vi "GetWinScale.vi"(8 "Error In":errorcluster, 11 "Window Name":string) -> (0 "Error Out":errorcluster, 3 "Scale":dbl)   [LabVIEW 2025]
uses:
  user32.dll
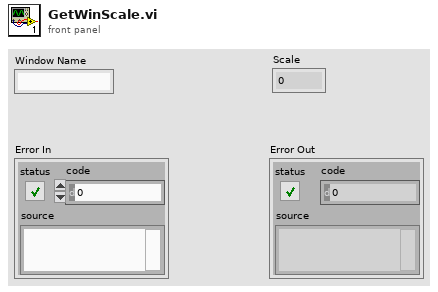
[diagram p1: front panel]
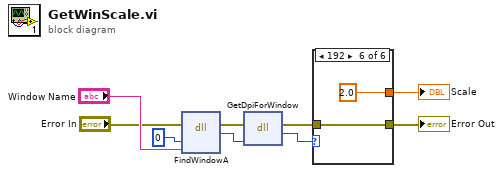
[diagram p0: block diagram]
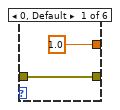
[diagram p2: hidden frame]
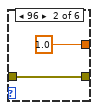
[diagram p3: hidden frame]
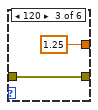
[diagram p4: hidden frame]
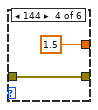
[diagram p5: hidden frame]
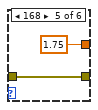
[diagram p6: hidden frame]
diagram:
  n1 = dll-call lib="User32.dll" fn="FindWindowA"(error in="Error In", "arg1"=0, "arg2"="Window Name") -> (error out=w6:errorcluster, "return type"=w9:i64)  [unwired: 3 in, 2 out]
  n2 = dll-call lib="User32.dll" fn="GetDpiForWindow" ("user32.dll:GetCursorPos")(error in=w6, "hWnd"=w9) -> (error out=w3:errorcluster, "return type"=w2:u32)  [unwired: 2 in, 2 out]
  n3 = case shown="192" w2 {
    tunnel: [w11 w13 w15 w17 w19 w21] -> w4
    tunnel: w3 -> [w11 w13 w15 w17 w19 w21]
    tunnel: [1.0 1.0 1.25 1.5 1.75 2.0] -> w1
    frame 0, Default {
    }
    frame 96 {
    }
    frame 120 {
    }
    frame 144 {
    }
    frame 168 {
    }
    frame 192 {
    }
  }
  "Error Out" <- w4
  "Scale" <- w1
